vi "U3 Frequency Measurement and Analog Input.vi"() -> ()   [LabVIEW 2021]
panel:
  out "Iteration":i32
  out "Frequency (FIO5)":dbl format="%.2f"
  out "Period (FIO5)":dbl format="%.6f"
  in  "error in":errorcluster
  in  "Address":string="1"
  in  "FirstFound":bool=TRUE
  in  "stop":bool
  out "Counter1 (FIO6)":u32
  out "error out":errorcluster
  out "Error Message":string
  out "AIN0-AIN3":dbl[](array[numeric]) format="%.6f"
  # "Timer clock is 1 MHz.\nFIO4 is 8-bit PWM output at 3906 Hz, with a 50% duty cycle.\nFIO5 is a 16-bit rising-to-rising edge measurement input.\nFIO6 is hardware counter 1.\nFor testing, connect jumpers from FIO4 to FIO5 to FIO6.\n\nShows that doing command/response analog input does not affect the timers and counters.\nEvery second, this VI measures the frequency of the PWM output (using a hardware\ncounter and edge-to-edge measurement), and then retrieves AIN0-AIN3\nten times."
  # "seconds"
  # "This VI passes a timer\nbase clock constant that\nis valid for hardware V1.21.\nFor hardware V1.20 change\nLJ_tc48MHZ_DIV to LJ_tc24MHZ_DIV."
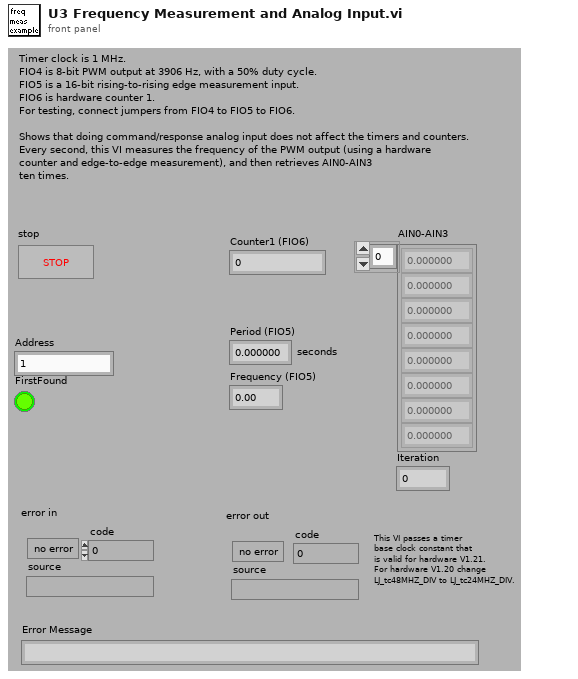
[diagram p1: front panel]
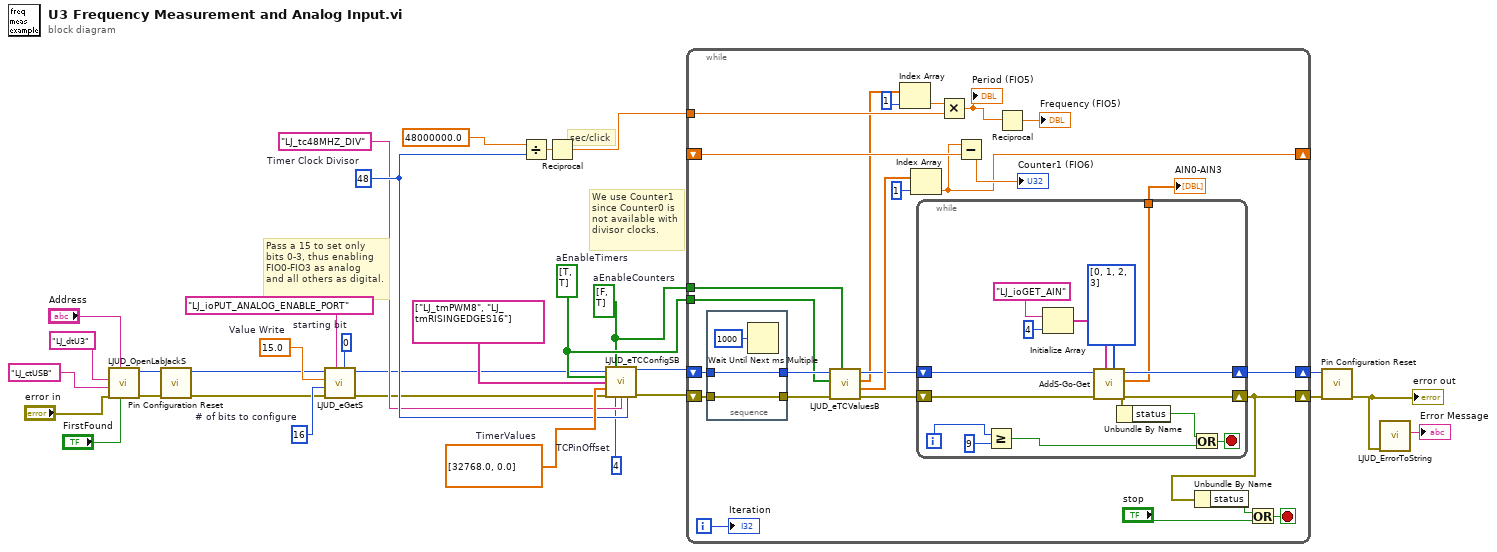
[diagram p0: block diagram]
diagram:
  w7 = 16  # # of bits to configure
  w9 = 0  # starting bit
  w10 = 15.0  # Value Write
  w11 = 4  # TCPinOffset
  w16 = bool[] [FALSE, TRUE]  # aEnableCounters
  w17 = bool[] [TRUE, TRUE]  # aEnableTimers
  w19 = 48  # Timer Clock Divisor
  w21 = dbl[] [32768.0, 0.0]  # TimerValues
  # "Pass a 15 to set only\nbits 0-3, thus enabling\nFIO0-FIO3 as analog\nand all others as digital."
  # "We use Counter1\nsince Counter0 is\nnot available with\ndivisor clocks."
  # "sec/click"
  n1 = call "LJUD_OpenLabJackS.vi"("FirstFound"="FirstFound", "Address"="Address", "error in"="error in", "ConnectionType"="LJ_ctUSB", "DeviceType"="LJ_dtU3") -> ("error out"=w5:errorcluster, "Handle"=w6:i32)  [unwired: 4 in, 1 out]
  n2 = call "Pin Configuration Reset.vi"("error in"=w5, "Handle In"=w6) -> ("error out"=w4:errorcluster, "Handle Out"=w3:i32)  [unwired: 8 in]
  n3 = call "LJUD_eGetS.vi"("Channel"=w9, "IOType"="LJ_ioPUT_ANALOG_ENABLE_PORT", "error in"=w4, "x1"=w7, "Value Write"=w10, "Handle In"=w3) -> ("error out"=w1:errorcluster, "Handle Out"=w2:i32)  [unwired: 3 in, 1 out]
  n4 = Divide(x=48000000.0, y=w19) -> (x/y=w26:dbl)
  n5 = Reciprocal(x=w26) -> (1/x=w25:dbl)
  n6 = call "LJUD_eTCConfigSB.vi"("Handle In"=w2, "aEnableCounters"=w16, "aEnableTimers"=w17, "aTimerModes"=string[] ["LJ_tmPWM8", "LJ_tmRISINGEDGES16"] ("TimerModes"), "aTimerValues"=w21, "error in"=w1, "TCPinOffset"=w11, "TimerClockBase"="LJ_tc48MHZ_DIV" ("Timer Clock Base"), "TimerClockDivisor"=w19) -> ("Handle Out"=w23:i32, "error out"=w22:errorcluster)  [unwired: 5 in]
  n7 = while {
    tunnel: w16 -> [w32]
    tunnel: w17 -> [w33]
    shift-left: _ -> [w40]
    shift-right: [w38] -> _
    tunnel: w25 -> [w43]
    shift-left: w22 -> [w54]
    shift-right: [w45] -> w14
    shift-left: w23 -> [w55]
    shift-right: [w56] -> w15
    i -> [w37]
    stop <- w47 stop-if-true
    n8 = stacked-sequence {
      tunnel: [w73] -> w49
      tunnel: [w72] -> w48
      tunnel: w55 -> [w73]
      tunnel: w54 -> [w72]
      frame #0 {
        n9 = Wait Until Next ms Multiple(millisecond multiple=u32 1000) -> ()  [unwired: 1 out]
      }
    }
    n10 = call "LJUD_eTCValuesB.vi"("aReadCounters"=w32, "error in"=w48, "aReadTimers"=w33, "Handle In"=w49) -> ("error out"=w51:errorcluster, "aCounterValues"=w53:dbl[], "aTimerValues Read"=w34:dbl[], "Handle Out"=w50:i32)  [unwired: 4 in]
    n11 = Index Array(array=w34, index=1 ("Index")) -> (element=w35:dbl)
    n12 = Index Array(array=w53, index=1 ("Index")) -> (element=w38:dbl)
    n13 = while {
      tunnel: [w61] -> w57
      shift-left: w51 -> [w70]
      shift-right: [w68] -> w45
      shift-left: w50 -> [w62]
      shift-right: [w69] -> w56
      i -> [w65]
      stop <- w67 stop-if-true
      n14 = Greater Or Equal?(x=w65, y=9) -> (x >= y?=w63:bool)
      n15 = Initialize Array("LJ_ioGET_AIN" ("IOType"), 4 ("Dimension Size")) -> (w58:string[])
      n16 = call "AddS-Go-Get.vi"("Channels"=i32[] [0, 1, 2, 3], "IOTypes"=w58, "error in"=w70, "Handle In"=w62) -> ("error out"=w68:errorcluster, "Values Read"=w61:dbl[], "Handle Out"=w69:i32)  [unwired: 5 in]
      n17 = Unbundle By Name(w68) -> ("status"=w66:bool)
      n18 = Or(x=w66, y=w63) -> (x .or. y?=w67:bool)
    }
    "AIN0-AIN3" <- w57
    n19 = Multiply(x=w35, y=w43) -> (x*y=w42:dbl)
    "Period (FIO5)" <- w42
    n20 = Subtract(x=w38, y=w40) -> (x-y=→"Counter1 (FIO6)":dbl)
    n21 = Reciprocal(x=w42) -> (1/x=→"Frequency (FIO5)":dbl)
    n22 = Unbundle By Name(w45) -> ("status"=w46:bool)
    n23 = Or(x=w46, y="stop") -> (x .or. y?=w47:bool)
    "Iteration" <- w37
  }
  n24 = call "Pin Configuration Reset.vi"("error in"=w14, "Handle In"=w15) -> ("error out"=w13:errorcluster)  [unwired: 8 in, 1 out]
  "error out" <- w13
  n25 = call "LJUD_ErrorToString.vi"("error in"=w13) -> ("String"=→"Error Message":string)  [unwired: 10 in]
